vi "Simple_DAQ_with_timing_loop.vi"() -> ()   [LabVIEW 2021]
panel:
  in  "Sample Rate (Hz)":dbl=2.0
  in  "See Log FilePath":bool
  out "Log File Name":string
  out "Log Date & Time":string
  out "Log File Path":path
  out "error out":errorcluster
  in  "Start Logging":bool
  out "Pressure Chart":dbl[](graph)
  out "Date & Time":string
  out "Pressure (Bar)":dbl format="%#2_4f"
  in  "Start Aquisition":bool
  out "Voltage Detected":dbl format="%0.2f"
  in  "Stop Button":bool
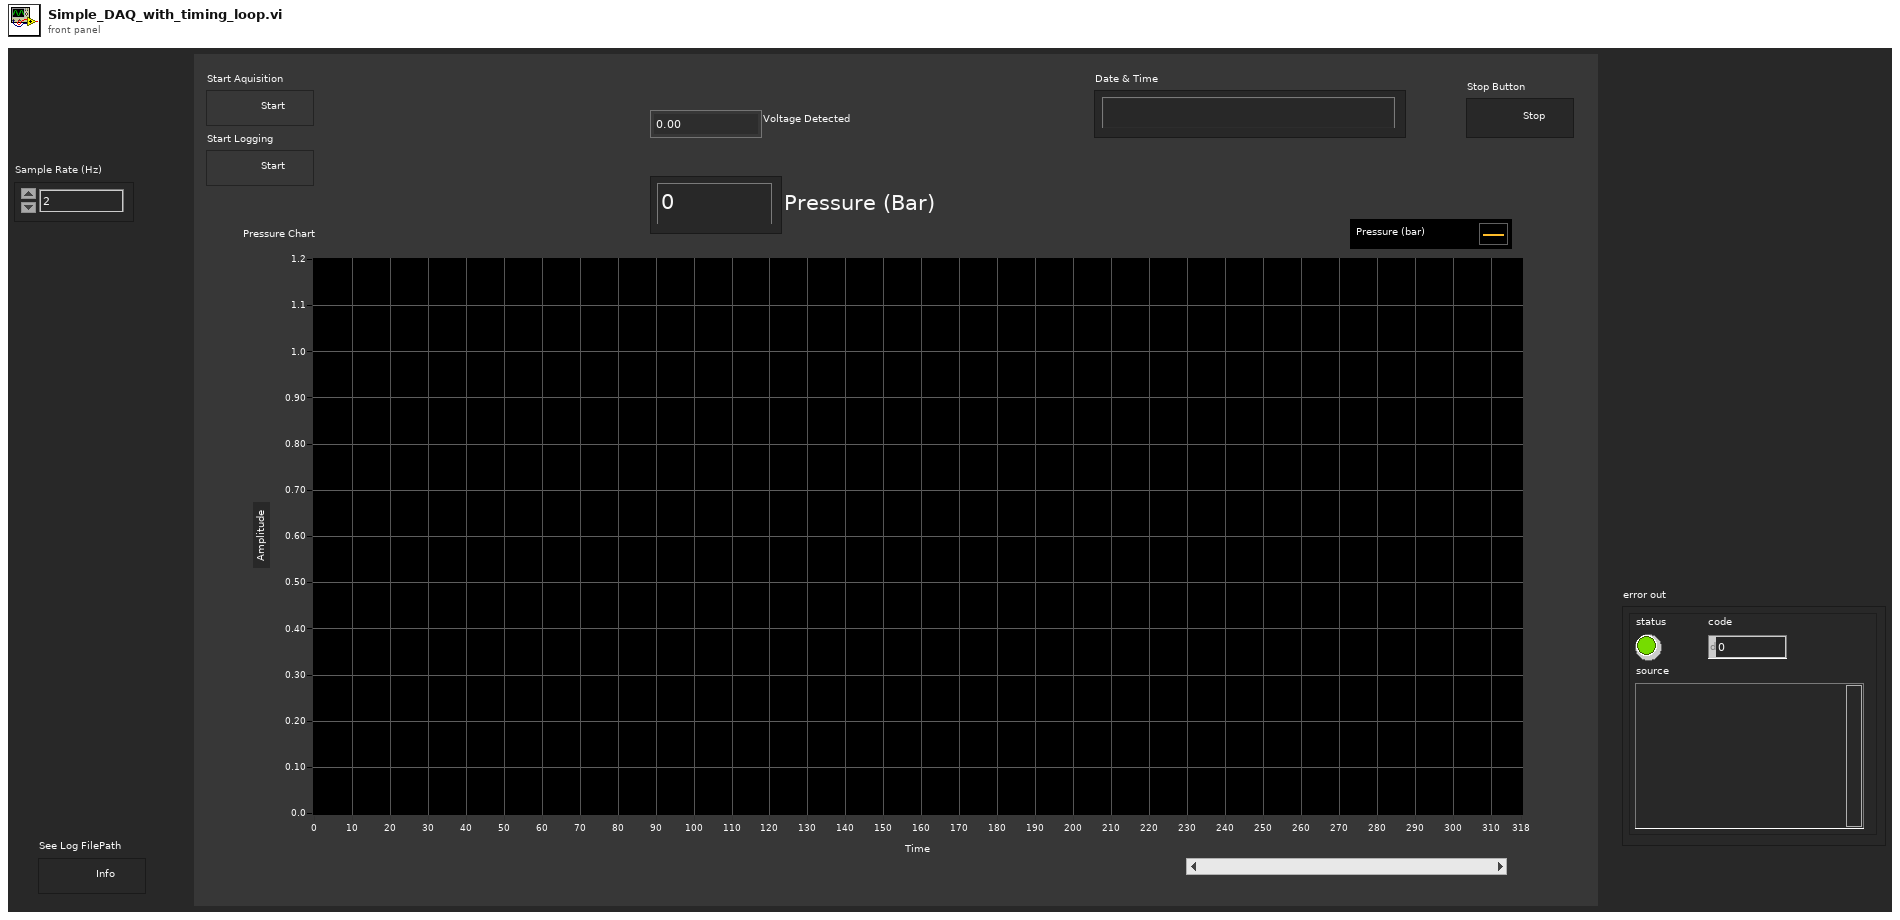
[diagram p1: front panel]
types:
  T1 = enum16{"open", "replace", "create", "open or create", "replace or create", "replace or create with confirmation"}
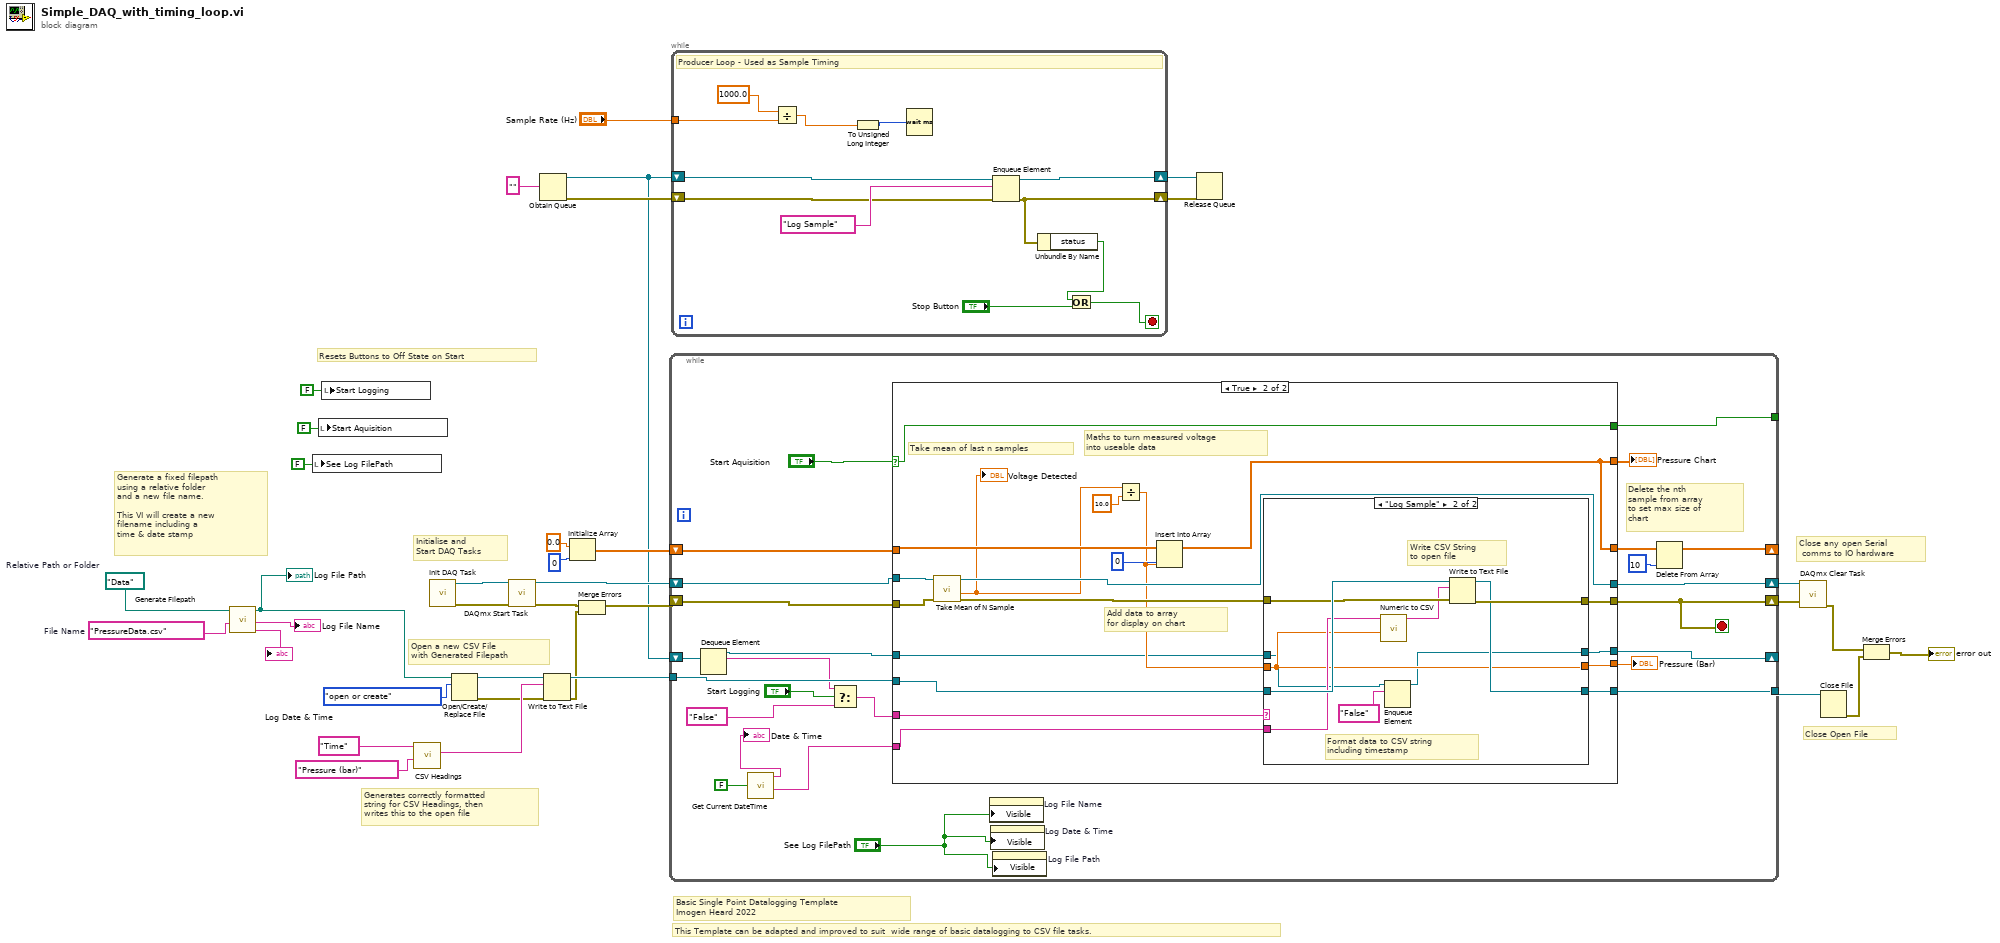
[diagram p0: block diagram]
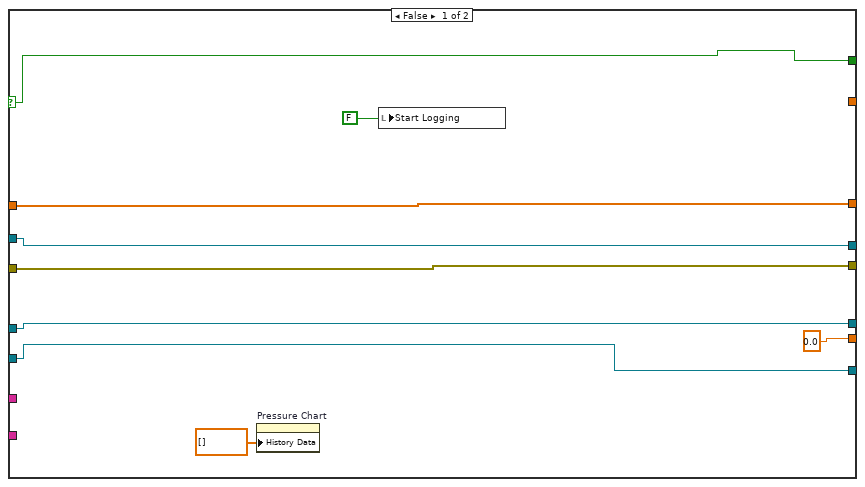
[diagram p2: hidden frame]
diagram:
  w25 = "PressureData.csv"  # File Name
  w26 = path "Data"  # Relative Path or Folder
  # "Close Open File"
  # "Close any open Serial\n comms to IO hardware"
  # "Generates correctly formatted\nstring for CSV Headings, then\nwrites this to the open file"
  # "Open a new CSV File\nwith Generated Filepath"
  # "Generate a fixed filepath\nusing a relative folder\nand a new file name.\n\nThis VI will create a new\nfilename including a\ntime & date stamp"
  # "This Template can be adapted and improved to suit  wide range of basic datalogging to CSV file tasks."
  # "Basic Single Point Datalogging Template\nImogen Heard 2022"
  # "Initialise and \nStart DAQ Tasks"
  # "Resets Buttons to Off State on Start"
  n1 = call "Generate Filepath.vi"("File Name"=w25, "Relative Path or Folder"=w26) -> ("Date & Time"=→"Log Date & Time":string, "Log File Name"=→"Log File Name":string, "File Path Output"=w21:path)  [unwired: 7 in]
  "Log File Path" <- w21
  n2 = local write "See Log FilePath"(FALSE ("See Log FilePath")) -> ()
  n3 = local write "Start Aquisition"(FALSE ("Start Aquisition")) -> ()
  n4 = local write "Start Logging"(FALSE ("Start Logging")) -> ()
  n5 = call "CSV Headings.vi"("Heading 2"="Pressure (bar)" ("element"), "Heading 1"="Time") -> ("CSV Heading String"=w11:string)  [unwired: 9 in]
  n6 = call "Init DAQ Task.vi"() -> ("error out"=w28:errorcluster, "Refnum out"=w36:refnum<k21>)  [unwired: 10 in]
  n7 = Open/Create/Replace File(file path (use dialog)=w21, operation (0:open)=T1."open or create") -> (refnum out=w20:refnum<file>, error out=w7:errorcluster)  [unwired: 4 in, 1 out]
  n8 = call <vilib>:"DAQmx Start Task.vi"("task/channels in"=w36, "error in"=w28) -> ("task out"=w35:refnum<k21>, "error out"=w23:errorcluster)  [unwired: 12 in]
  n9 = Obtain Queue(element data type="" ("element")) -> (queue out=w3:refnum<queue>, error out=w5:errorcluster)  [unwired: 4 in, 1 out]
  n10 = Write to Text File(file (use dialog)=w20, text=w11, error in=w7) -> (refnum out=w19:refnum<file>, error out=w18:errorcluster)  [unwired: 1 in, 1 out]
  n11 = Initialize Array(0.0 ("y"), 0 ("dimension size")) -> (w32:dbl[])
  n12 = Merge Errors(w23, w18) -> (w24:errorcluster)
  n13 = while {
    shift-right: [w59] -> w34
    shift-left: w35 -> [w61]
    shift-right: [w42] -> w16
    shift-left: w24 -> [w60]
    shift-right: [w54] -> _
    shift-left: w32 -> [w58]
    tunnel: [w52] -> w17
    tunnel: w19 -> [w50]
    tunnel: [w47] -> _
    shift-right: [w37] -> _
    shift-left: w3 -> [w43]
    stop <- w42 stop-if-true
    # "Delete the nth\nsample from array\nto set max size of \nchart"
    n14 = Dequeue Element(queue=w43) -> (queue out=w38:refnum<queue>, element=w41:string)  [unwired: 2 in, 2 out]
    n15 = call "Get Current DateTime.vi"("Leading Apostrophe"=FALSE) -> ("Time String"=w49:string, "Date/Time String"=→"Date & Time":string)  [unwired: 7 in, 2 out]
    n16 = Select(t=w41, s="Start Logging", f="False") -> (s? t:f=w39:string)
    n17 = case shown="True" "Start Aquisition" {
      selector: "Start Aquisition" -> [w63 w75]
      tunnel: w61 -> [w70 w88]
      tunnel: w60 -> [w69 w89]
      tunnel: [w69 w82] -> w42
      tunnel: [w70 w81] -> w59
      tunnel: w58 -> [w67 w85]
      tunnel: [w67 w84] -> w55
      tunnel: [0.0 w79] -> w53
      tunnel: [_ w84] -> w57
      tunnel: w50 -> [w65 w78]
      tunnel: [w65 w77] -> w52
      tunnel: w49 -> [_ w76]
      tunnel: [w63 w75] -> w47
      tunnel: w39 -> [_ w74]
      tunnel: w38 -> [w62 w73]
      tunnel: [w62 w72] -> w37
      frame False {
        n18 = property on="Pressure Chart" class="WFChart (strict)"("History Data"=dbl[] []) -> ()  [unwired: 2 in, 2 out]
        n19 = local write "Start Logging"(FALSE ("Start Aquisition")) -> ()
      }
      frame True {
        # "Add data to array\nfor display on chart"
        # "Maths to turn measured voltage\ninto useable data"
        # "Take mean of last n samples"
        n20 = call "Take Mean of N Sample.vi"("error in (no error)"=w89, "Refnum in"=w88) -> ("error out"=w83:errorcluster, "Mean Voltage Detected"=w71:dbl, "Refnum out"=w81:refnum<k21>)  [unwired: 7 in]
        "Voltage Detected" <- w71
        n21 = Divide(x=w71, y=10.0) -> (x/y=w80:dbl)
        n22 = Insert Into Array(array=w85, index=0, new element=w80) -> (w84:dbl[])
        n23 = case shown="\"Log Sample\"" w74 {
          tunnel: w83 -> [w93 w102]
          tunnel: [w93 w101] -> w82
          tunnel: w80 -> [w92 w97]
          tunnel: [w92 w97] -> w79
          tunnel: w78 -> [w91 w103]
          tunnel: [w91 w100] -> w77
          tunnel: w76 -> [_ w98]
          tunnel: w73 -> [w90 w96]
          tunnel: [w90 w95] -> w72
          frame "False", Default {
          }
          frame "Log Sample" {
            # "Write CSV String\nto open file"
            # "Format data to CSV string\nincluding timestamp"
            n24 = call "Numeric to CSV.vi"("Numeric"=w97, "Time String"=w98) -> ("spreadsheet string"=w99:string)  [unwired: 9 in]
            n25 = Enqueue Element(queue=w96, element="False") -> (queue out=w95:refnum<queue>)  [unwired: 2 in, 2 out]
            n26 = Write to Text File(file (use dialog)=w103, text=w99, error in=w102) -> (refnum out=w100:refnum<file>, error out=w101:errorcluster)  [unwired: 1 in, 1 out]
          }
        }
      }
    }
    "Pressure Chart" <- w57
    "Pressure (Bar)" <- w53
    n27 = property on="Log File Name" class="Str"("Visible"="See Log FilePath") -> ()  [unwired: 2 in, 2 out]
    n28 = property on="Log Date & Time" class="Str"("Visible"="See Log FilePath") -> ()  [unwired: 2 in, 2 out]
    n29 = property on="Log File Path" class="Path"("Visible"="See Log FilePath") -> ()  [unwired: 2 in, 2 out]
    n30 = Delete From Array(array=w55, index=10) -> (array with subset deleted=w54:dbl[])  [unwired: 1 in, 1 out]
  }
  n31 = while {
    shift-right: [w114] -> w6
    shift-left: w3 -> [w115]
    shift-right: [w111] -> w4
    shift-left: w5 -> [w112]
    tunnel: "Sample Rate (Hz)" -> [w107]
    stop <- w109 stop-if-true
    # "Producer Loop - Used as Sample Timing"
    n32 = Divide(x=1000.0, y=w107) -> (x/y=w104:dbl)
    n33 = To Unsigned Long Integer(number=w104) -> (unsigned 32bit integer=w105:u32)
    n34 = Wait (ms)(milliseconds to wait=w105) -> ()  [unwired: 1 out]
    n35 = Enqueue Element(queue=w115, element="Log Sample", error in (no error)=w112) -> (queue out=w114:refnum<queue>, error out=w111:errorcluster)  [unwired: 1 in, 1 out]
    n36 = Unbundle By Name(w111) -> ("status"=w110:bool)
    n37 = Or(x=w110, y="Stop Button") -> (x .or. y?=w109:bool)
  }
  n38 = Release Queue(queue=w6, error in (no error)=w4) -> ()  [unwired: 1 in, 3 out]
  n39 = call <vilib>:"DAQmx Clear Task.vi"("task in"=w34, "error in"=w16) -> ("error out"=w14:errorcluster)  [unwired: 13 in]
  n40 = Close File(refnum=w17) -> (error out=w13:errorcluster)  [unwired: 1 in, 1 out]
  n41 = Merge Errors(w14, w13) -> (→"error out":errorcluster)
